vi "FourCornerAntennaAlignment_.vi"(10 "Y corners, 7, 0, 63, 56":dbl[](array[numeric])=[144.21, 145.21, 338.21, 339.2] format="%.4f", 11 "X corners, 7, 0, 63, 56":dbl[](array[numeric])=[204.42, 398.3, 203.44, 397.44] format="%.4f") -> (0 "Valid Readings":bool, 1 "x angle all":dbl, 3 "x direction angle":dbl format="%.4f")   [LabVIEW 2018]
doc: "uses motion controller coordinates of the four corner crosshairs of the antenna to compute the angle that the antenna is rotated wrt to the x y axes of the motion system.\n\nThe original module/antenna numbers were flipped in 3/2018. The calculation is the same but the module numbers were re-assigned."
uses:
  <vilib>/Analysis/baseanly.llb/Mean (DBL).vi
  <vilib>/Analysis/NI_AALBase.lvlib
panel:
  out "degrees 2":dbl[](array[numeric])
  out "standard deviation":dbl format="%.5f"
  out "y direction angle":dbl format="%.4f"
  out "degrees":dbl[](array[numeric])
  # "could drop points outside the sdev\n\nor\n\ntake the two x direction computations - doing this for now"
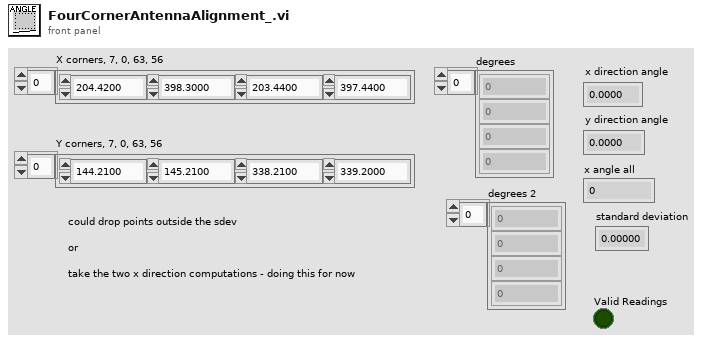
[diagram p1: front panel]
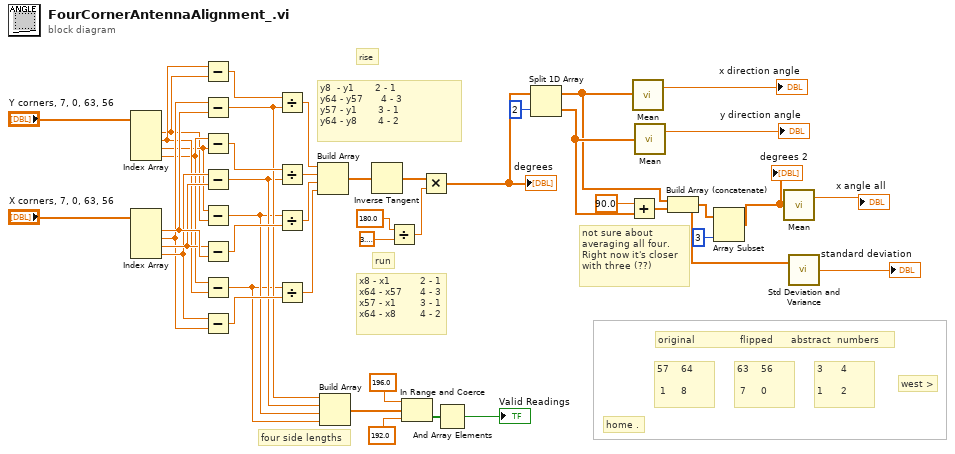
[diagram p0: block diagram]
diagram:
  # "four side lengths"
  # "not sure about\naveraging all four.\nRight now it's closer\nwith three (??)"
  # "original               flipped      abstract  numbers"
  # "west >"
  # "home ."
  # "3      4\n\n1      2"
  # "63    56\n\n 7     0"
  # "57    64\n\n 1     8"
  # "y8  - y1       2 - 1\ny64 - y57      4 - 3\ny57 - y1       3 - 1\ny64 - y8       4 - 2"
  # "x8 - x1          2 - 1\nx64 - x57      4 - 3\nx57 - x1        3 - 1\nx64 - x8        4 - 2"
  # "rise"
  # "run"
  n1 = Index Array(array="Y corners, 7, 0, 63, 56") -> (element #1=w33:dbl, element #2=w36:dbl, element #3=w34:dbl, element #4=w35:dbl)  [unwired: 4 in]
  n2 = Index Array(array="X corners, 7, 0, 63, 56") -> (element #1=w40:dbl, element #2=w37:dbl, element #3=w39:dbl, element #4=w38:dbl)  [unwired: 4 in]
  n3 = Subtract(x=w36, y=w33) -> (x-y=w31:dbl)
  n4 = Subtract(x=w37, y=w40) -> (x-y=w9:dbl)
  n5 = Subtract(x=w35, y=w34) -> (x-y=w30:dbl)
  n6 = Subtract(x=w38, y=w39) -> (x-y=w8:dbl)
  n7 = Subtract(x=w34, y=w33) -> (x-y=w7:dbl)
  n8 = Subtract(x=w39, y=w40) -> (x-y=w29:dbl)
  n9 = Subtract(x=w35, y=w36) -> (x-y=w6:dbl)
  n10 = Subtract(x=w38, y=w37) -> (x-y=w28:dbl)
  n11 = Divide(x=w31, y=w9) -> (x/y=w27:dbl)
  n12 = Divide(x=w30, y=w8) -> (x/y=w26:dbl)
  n13 = Divide(x=w7, y=w29) -> (x/y=w25:dbl)
  n14 = Divide(x=w6, y=w28) -> (x/y=w24:dbl)
  n15 = Build Array(w27, w26, w25, w24) -> (w23:dbl[])
  n16 = Build Array(w9, w8, w7, w6) -> (w5:dbl[])
  n17 = Inverse Tangent(1:w23) -> (0:w41:dbl[])
  n18 = Divide(x=180.0 ("y"), y=3.141592653589793) -> (x/y=w44:dbl)
  n19 = In Range and Coerce(upper limit=196.0 ("y"), x=w5, lower limit=192.0 ("y")) -> (In Range?=w2:bool[])  [unwired: 1 out]
  n20 = Multiply(x=w41, y=w44) -> (x*y=w22:dbl[])
  "degrees" <- w22
  n21 = And Array Elements(Boolean array=w2) -> (logical AND=→"Valid Readings":bool)
  n22 = Split 1D Array(array=w22, index=2) -> (first subarray=w15:dbl[], second subarray=w17:dbl[])
  n23 = Add(x=90.0, y=w17) -> (x+y=w16:dbl[])
  n24 = call-poly <vilib>:"Mean.vi"("X"=w15) -> ("mean"=→"x direction angle":dbl)  [unwired: 1 out]
  n25 = call-poly <vilib>:"Mean.vi"("X"=w17) -> ("mean"=→"y direction angle":dbl)  [unwired: 1 out]
  n26 = Build Array (concatenate)(w15, w16) -> (w12:dbl[])
  n27 = Array Subset(array=w12, length=3) -> (w10:dbl[])  [unwired: 1 in]
  "degrees 2" <- w10
  n28 = call-poly <vilib>:"Mean.vi"("X"=w10) -> ("mean"=→"x angle all":dbl)  [unwired: 1 out]
  n29 = call <vilib>:"Std Deviation and Variance.vi"("X"=w12) -> ("standard deviation"=→"standard deviation":dbl)  [unwired: 1 in, 2 out]
